vi "Threshold_hysteresis.vi"(1 "Range":dbl, 2 "Threshold":dbl, 3 "X":dbl) -> (0 "Threshold_State":T1)   [LabVIEW 2019]
uses:
  TypeDefs/Hysteresis_State.ctl
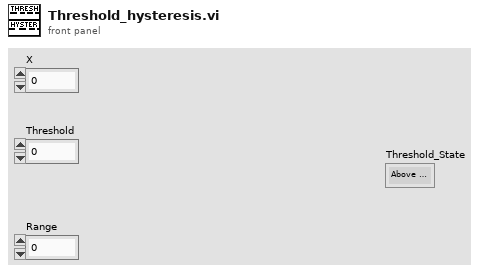
[diagram p1: front panel]
types:
  T1 = typedef "Hysteresis_State.ctl" = enum16{"Above Threshold", "Below Threshold"}
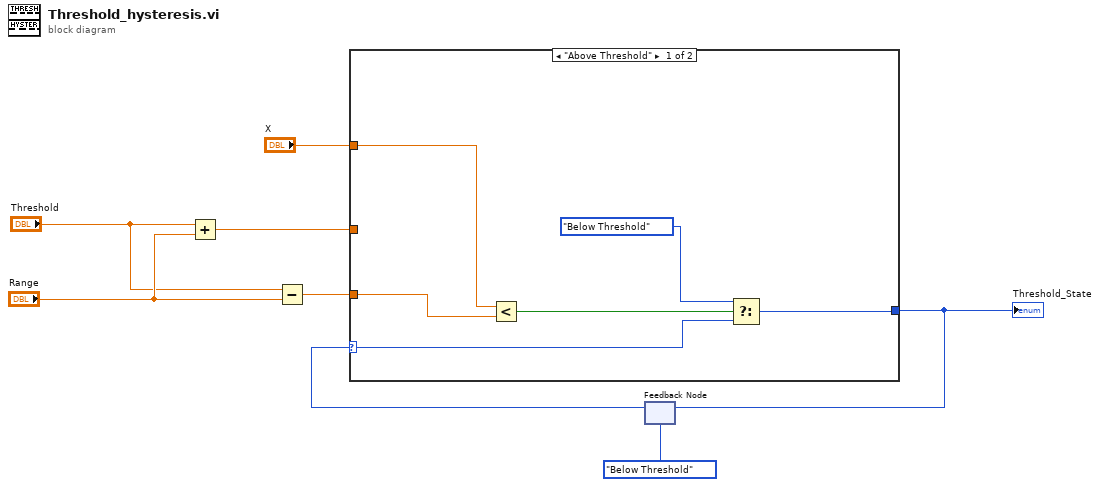
[diagram p0: block diagram]
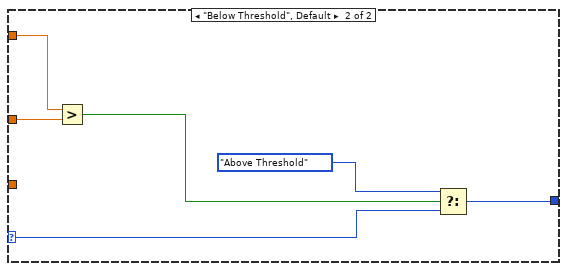
[diagram p2: hidden frame]
diagram:
  n1 = Add(x="Threshold", y="Range") -> (x+y=w4:dbl)
  n2 = Subtract(x="Threshold", y="Range") -> (x-y=w2:dbl)
  n3 = feedback #1(Hysteresis_State."Below Threshold") -> (w5:T1)
  n4 = case shown="\"Above Threshold\"" w5 {
    selector: w5 -> [w9 w20]
    tunnel: [w14 w19] -> w1
    tunnel: w4 -> [_ w17]
    tunnel: "X" -> [w11 w18]
    tunnel: w2 -> [w10 _]
    frame "Above Threshold" {
      n5 = Less?(x=w11, y=w10) -> (x < y?=w12:bool)
      n6 = Select(t=Hysteresis_State."Below Threshold", s=w12, f=w9) -> (s? t:f=w14:T1)
    }
    frame "Below Threshold", Default {
      n7 = Greater?(x=w18, y=w17) -> (0:w16:bool)
      n8 = Select(t=Hysteresis_State."Above Threshold", s=w16, f=w20) -> (s? t:f=w19:T1)
    }
  }
  "Threshold_State" <- w1
  n9 = feedback-in #1(w1) -> ()
